vi "Display merged still images.vi"(0 "Image colors":u32[](array[colorbox])=[16711680, 1048329], 3 "Image info":T3(array[cluster])=[{"File name"=path "\\\\jg-i\\c-drive/LabView development/Glimpse/Test Data/Merge test/gelles00096full.tif", "TIFF stack?"=TRUE, "Frame # if stack?"=1}, {"File name"=path "\\\\jg-i\\c-drive/LabView development/Glimpse/Test Data/Merge test/gelles00097full.tif", "TIFF stack?"=TRUE, "Frame # if stack?"=1}], 5 "Transform":u16(ring) items=["linear conformal", "affine", "projective"]) -> (1 "ROI Out":i32[](array[numeric]), 4 "Transform out":u16(ring) items=["linear conformal", "affine", "projective"], 6 "Image info Out":T3(array[cluster])=[{"File name"=path "\\\\jg-i\\c-drive/LabView development/Glimpse/Test Data/Merge test/gelles00096full.tif", "TIFF stack?"=TRUE, "Frame # if stack?"=1}, {"File name"=path "\\\\jg-i\\c-drive/LabView development/Glimpse/Test Data/Merge test/gelles00097full.tif", "TIFF stack?"=TRUE, "Frame # if stack?"=1}], 7 "Display info out":T2(array[cluster]), 8 "Image colors out":u32[](array[colorbox])=[16711680, 1048329])   [LabVIEW 2011]
doc: "Allows the user to select two still images (individual tiffs or frames from a stack) and adust their black/white levels while displaying a pseudocolor merged image. Merged image can optionally be saved as a JPEG file."
uses:
  <vilib>/vision/Image Controls.llb/IMAQ Image.ctl
  GLIMPSE Globals.vi
panel:
  in  "Crop":bool
  in  "Remove\nCrop":bool
  in  "Save\nMerged Image":bool
  in  "Write text overlay":bool=TRUE
  in  "stop":bool
  in  "Load\nimages":bool
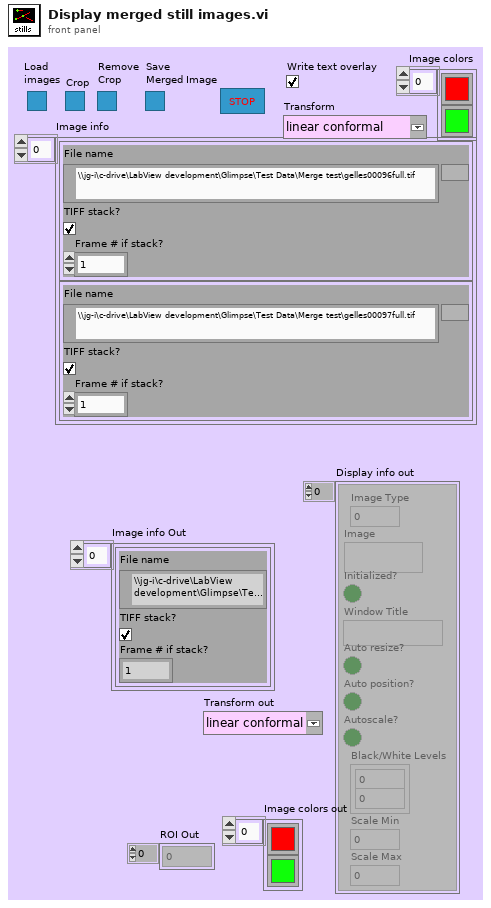
[diagram p1: front panel]
types:
  T1 = typedef "IMAQ Image.ctl" = refnum<image>
  T2 = cluster{"Image Type":u32, "Image":T1, "Initialized?":bool, "Window Title":string, "Auto resize?":bool, "Auto position?":bool, "Autoscale?":bool, "Black/White Levels":cluster{ext, ext}, "Scale Min":ext, "Scale Max":ext}[]
  T3 = cluster{"File name":path, "TIFF stack?":bool, "Frame # if stack?":u32}[]
  T4 = typedef "ROI Descriptor" = cluster{"Global Rectangle":i32[], "Contours":cluster{"ID":enum32{"External", "Internal"}, "Type":u32, "Coordinates":i32[]}[]}
  T5 = enum32{"existing file", "new file", "new or existing file", "existing dir", "new dir", "new or existing dir", "existing file (use LLBs)", "new file (use LLBs)", "new or existing file (use LLBs)", "new or existing file or directory (use LLBs)"}
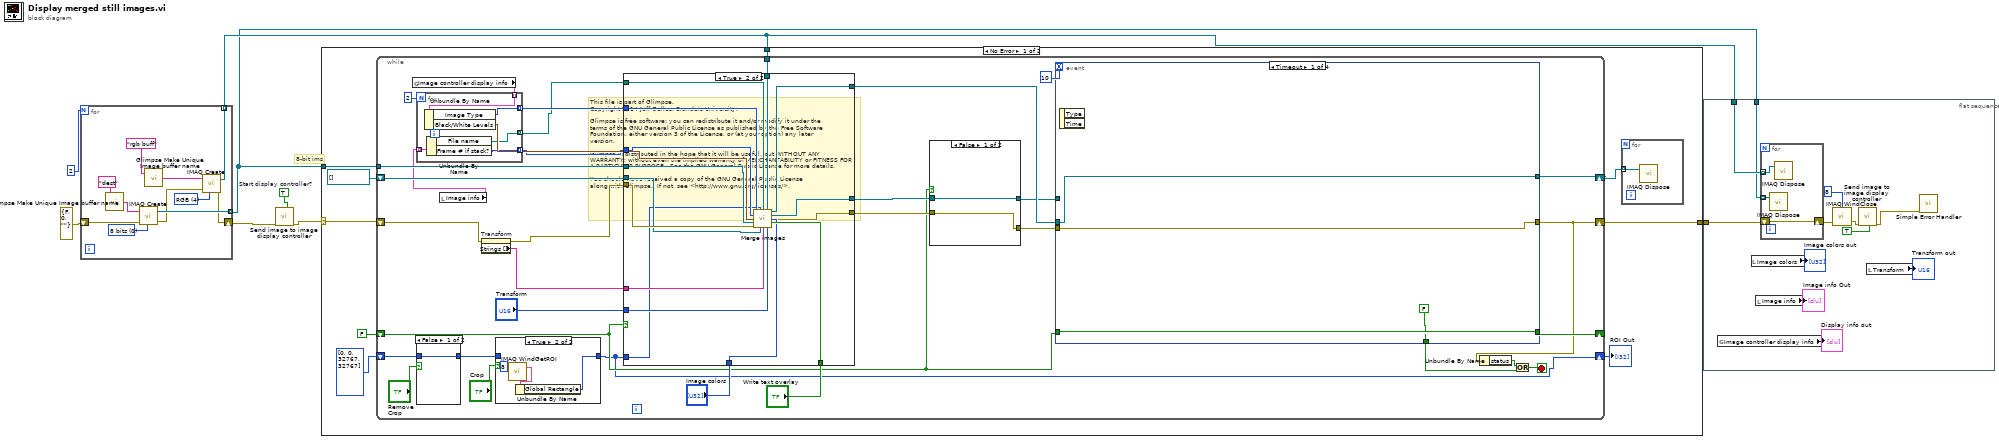
[diagram p0: block diagram]
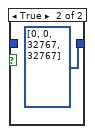
[diagram p3: hidden frame]
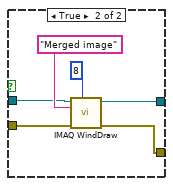
[diagram p4: hidden frame]
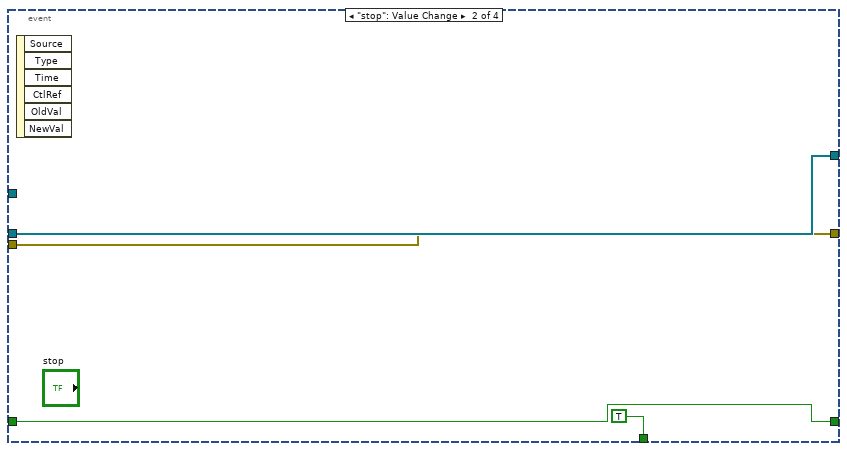
[diagram p6: hidden frame]
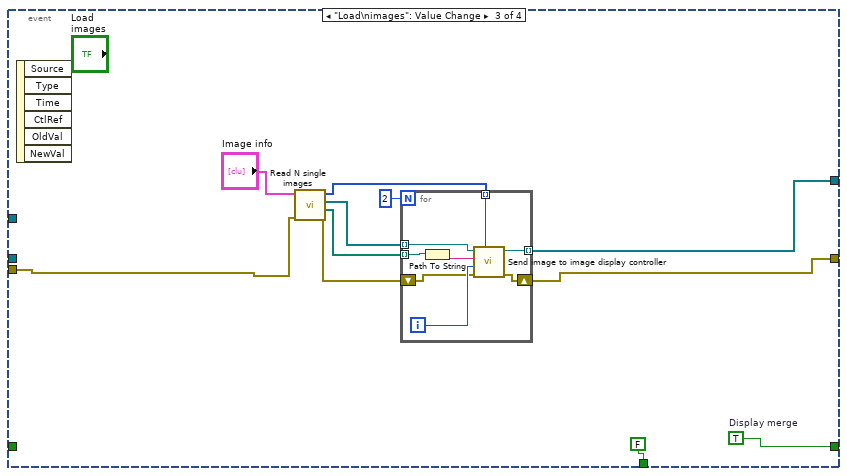
[diagram p7: hidden frame]
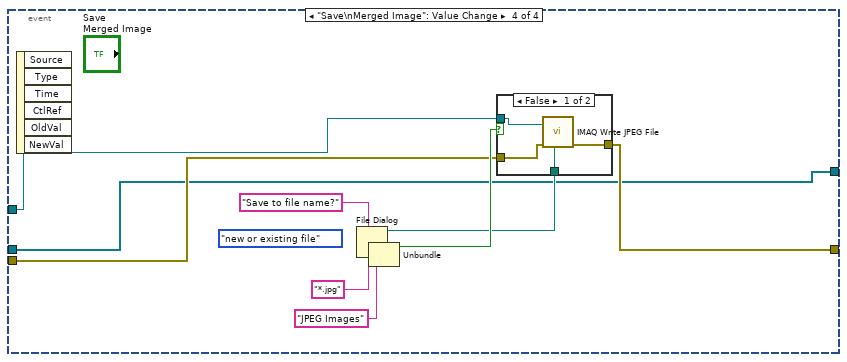
[diagram p8: hidden frame]
diagram:
  w8 = TRUE  # Start display controller?
  # "This file is part of Glimpse. \nCopyright 2014 Jeff Gelles, Brandeis University.    \n\nGlimpse is free software: you can redistribute it and/or modify it under the \nterms of the GNU General Public License as published by the Free Software \nFoundation, either version 3 of the License, or (at your option) any later \nversion.\n\nGlimpse is distributed in the hope that it will be useful, but WITHOUT ANY \nWARRANTY; without even the implied warranty of MERCHANTABILITY or FITNESS FOR \nA PARTICULAR PURPOSE.  See the GNU General Public License for more details.\n\nYou should have received a copy of the GNU General Public License\nalong with Glimpse.  If not, see <http://www.gnu.org/licenses/>."
  # "8-bit ims"
  n1 = for {
    N: 2 -> [_]
    shift-right: [w9] -> w4
    shift-left: errorcluster {"status"=FALSE, "code"=0, "source"=""} ("error out") -> [w16]
    tunnel: [w15] -> w1 mode=indexing
    tunnel: [w13] -> w3 mode=indexing
    w14 = u32 4 items=["8 bits", "16 bits", "Float", "Complex", "RGB", "HSL"] ("Image Type")
    w17 = u32 0 items=["8 bits", "16 bits", "Float", "Complex", "RGB", "HSL"] ("Image Type")
    n2 = call "Glimpse Make Unique Image buffer name.vi"("Buffer  base name"="dest") -> ("Image Name"=w19:string)  [unwired: 1 out]
    n3 = call "IMAQ Create"("Image Name"=w19, "Image Type"=w17, "error in (no error)"=w16) -> ("New Image"=w15:T1, "error out"=w10:errorcluster)  [unwired: 1 in, 1 out]
    n4 = call "Glimpse Make Unique Image buffer name.vi"("Buffer  base name"="rgb buff" ("Image Name")) -> ("Image Name"=w11:string)  [unwired: 1 out]
    n5 = call "IMAQ Create"("Image Name"=w11, "Image Type"=w14, "error in (no error)"=w10) -> ("New Image"=w13:T1, "error out"=w9:errorcluster)  [unwired: 1 in, 1 out]
  }
  n6 = call "Send image to image display controller.vi"("error in"=w4, "Start display controller?"=w8) -> ("error out"=w7:errorcluster)  [unwired: 5 in, 3 out]
  n7 = case shown="No Error" w7 {
    selector: w7 -> [w27 _]
    tunnel: w1 -> [w26 _]
    tunnel: w3 -> [w25 _]
    tunnel: [w23 _] -> w2
    frame No Error {
      n8 = while {
        shift-right: [w63] -> _
        shift-left: FALSE ("Display merge") -> [w40]
        shift-right: [w57] -> w23
        shift-left: w27 -> [w37]
        tunnel: w26 -> [w62]
        shift-right: [w61] -> w24
        shift-left: T1[] [] -> [w60]
        tunnel: w25 -> [w59]
        shift-right: [w30] -> w20
        shift-left: i32[] [0, 0, 32767, 32767] ("ROI") -> [w32]
        stop <- w54 stop-if-true
        n9 = global read "GLIMPSE Globals.vi" "Image controller display info"() -> (w51:T2)
        n10 = case shown="False" "Remove\nCrop" {
          tunnel: w32 -> [w68 _]
          tunnel: [w68 i32[] [0, 0, 32767, 32767] ("ROI")] -> w31
          frame False {
          }
          frame True {
          }
        }
        n11 = local read "Image info"() -> (w47:T3)
        n12 = for {
          N: 2 -> [_]
          tunnel: w51 -> [w83] mode=indexing
          tunnel: [w82] -> w50 mode=indexing
          tunnel: [w81] -> w48 mode=indexing
          tunnel: [w78] -> w49 mode=indexing
          tunnel: w47 -> [w80] mode=indexing
          tunnel: [w79] -> w46 mode=indexing
          n13 = Unbundle By Name(w83) -> ("Image Type"=w82:u32, "Black/White Levels"=w81:cluster{ext, ext})
          n14 = Unbundle By Name(w80) -> ("File name"=w78:path, "Frame # if stack?"=w79:u32)
        }
        n15 = property on="Transform" class="Ring (strict)"(error in=w37) -> (error out=w36:errorcluster, "Strings []"=w38:string[])  [unwired: 1 in, 1 out]
        n16 = case shown="True" "Crop" {
          tunnel: w31 -> [w64 _]
          tunnel: [w64 w65] -> w30
          frame False {
          }
          frame True {
            n17 = call "IMAQ WindGetROI"("Window Number (0...15)"=8) -> ("ROI Descriptor"=w67:T4)  [unwired: 1 in, 4 out]
            n18 = Unbundle By Name(w67) -> ("Global Rectangle"=w65:i32[])
          }
        }
        n19 = case shown="True" w40 {
          tunnel: w62 -> [_ w101]
          tunnel: w36 -> [w84 w100]
          tunnel: w60 -> [w85 w99]
          tunnel: w59 -> [_ w98]
          tunnel: [w84 w90] -> w43
          tunnel: [w85 w97] -> w58
          tunnel: w50 -> [_ w96]
          tunnel: w48 -> [_ w95]
          tunnel: w49 -> [_ w94]
          tunnel: w46 -> [_ w93]
          tunnel: "Write text overlay" -> [_ w92]
          tunnel: "Image colors" -> [_ w91]
          tunnel: [_ w89] -> w41
          tunnel: "Transform" -> [_ w88]
          tunnel: w38 -> [_ w87]
          tunnel: w30 -> [_ w86]
          frame False {
          }
          frame True {
            n20 = call "Merge images.vi"("Image types"=w96, "ROI"=w86, "File paths"=w94, "RGB image buffers in"=w98, "Overlay frame numbers"=w93, "Black/white levels"=w95, "8 bit scratch images"=w101, "Write text overlay?"=w92, "error in"=w100, "N-bit images in"=w99, "Transform types"=w87, "Transform number?"=w88, "Image colors"=w91) -> ("N-bit images out"=w97:T1[], "RGB Image out"=w89:T1, "error out"=w90:errorcluster)
          }
        }
        n21 = case shown="False" w40 {
          tunnel: w43 -> [w71 w75]
          tunnel: [w71 w74] -> w42
          tunnel: w41 -> [w70 w73]
          tunnel: [w70 w72] -> w35
          frame False {
          }
          frame True {
            n22 = call "IMAQ WindDraw"("Window Number (0...15)"=8, "error in (no error)"=w75, "Title"="Merged image", "Image"=w73) -> ("error out"=w74:errorcluster, "Image Out (duplicate)"=w72:T1)  [unwired: 2 in, 4 out]
          }
        }
        n23 = event shown="[0] Timeout" {
          selector: _ -> [_ _ _ _]
          dyn-events: _ -> [_ _ _ _]
          timeout: 10 -> [_ _ _ _]
          tunnel: [w104 w106 w115 _] -> w63
          tunnel: w40 -> [w104 w106 _ _]
          tunnel: [w105 w108 w114 w130] -> w61
          tunnel: w58 -> [w105 w108 _ w130]
          tunnel: [w103 w107 w110 w131] -> w57
          tunnel: w42 -> [w103 w107 w111 w132]
          tunnel: [FALSE TRUE FALSE _] -> w55
          tunnel: w35 -> [_ _ _ w133]
          event Timeout {
            n24 = event-data() -> ()  [unwired: 3 out]
          }
          event "stop": Value Change {
            n25 = event-data() -> ()  [unwired: 7 out]
          }
          event "Load\nimages": Value Change {
            w115 = TRUE  # Display merge
            n26 = event-data() -> ()  [unwired: 7 out]
            n27 = call "Read N single images.vi"("error in"=w111, "Image info"="Image info") -> ("error out"=w119:errorcluster, "File paths out"=w118:path[], "Images out"=w117:T1[], "Image types out"=w116:u32[])  [unwired: 4 out]
            n28 = for {
              N: 2 -> [_]
              tunnel: [w127] -> w114 mode=indexing
              shift-right: [w126] -> w110
              shift-left: w119 -> [w122]
              tunnel: w118 -> [w124] mode=indexing
              tunnel: w117 -> [w123] mode=indexing
              tunnel: w116 -> [w121] mode=indexing
              i -> [w125]
              n29 = Path To String(path=w124) -> (string=w128:string)
              n30 = call "Send image to image display controller.vi"("Image"=w123, "Window Title"=w128, "Window Number"=w125, "error in"=w122, "Image Type"=w121) -> ("Image Out"=w127:T1, "error out"=w126:errorcluster)  [unwired: 2 in, 2 out]
            }
          }
          event "Save\nMerged Image": Value Change {
            (unwired) T5."new or existing file" ("select mode (2)")
            n31 = event-data() -> ()  [unwired: 7 out]
            n32 = File Dialog(4:"JPEG Images" ("pattern label"), 6:"*.jpg" ("pattern"), 7:"Save to file name?" ("prompt")) -> (0:w129:errorcluster, 1:w138:bool, 3:w137:path)  [unwired: 1 in, 4 out]
            n33 = Unbundle(w129) -> ()  [unwired: 3 out]
            n34 = case shown="False" w138 {
              tunnel: [w142 w143] -> w131
              tunnel: w132 -> [w141 w143]
              tunnel: w137 -> [w140 _]
              tunnel: w133 -> [w139 _]
              frame False {
                n35 = call "IMAQ Write JPEG File"("error in (no error)"=w141, "File Path"=w140, "Image"=w139) -> ("error out"=w142:errorcluster)  [unwired: 2 in, 3 out]
              }
              frame True {
              }
            }
          }
        }
        n36 = Unbundle By Name(w57) -> ("status"=w56:bool)
        n37 = Or(x=w56, y=w55) -> (x .or. y?=w54:bool)
      }
      "ROI Out" <- w20
      n38 = for {
        tunnel: w24 -> [w29] mode=indexing
        n39 = call "IMAQ Dispose"("Image"=w29) -> ()  [unwired: 2 in, 4 out]
      }
    }
    frame Error {
    }
  }
  n40 = flat-sequence {
    tunnel: w3 -> [w155]
    tunnel: w2 -> [w154]
    tunnel: w1 -> [w153]
    frame #0 {
      n41 = global read "GLIMPSE Globals.vi" "Image controller display info"() -> (→"Display info out":T2)
      n42 = local read "Image colors"() -> (→"Image colors out":u32[])
      n43 = local read "Image info"() -> (→"Image info Out":T3)
      n44 = for {
        tunnel: w155 -> [w157] mode=indexing
        shift-right: [w158] -> w152
        shift-left: w154 -> [w158]
        tunnel: w153 -> [w156] mode=indexing
        n45 = call "IMAQ Dispose"("Image"=w156) -> ()  [unwired: 2 in, 4 out]
        n46 = call "IMAQ Dispose"("Image"=w157) -> ()  [unwired: 2 in, 4 out]
      }
      n47 = call "IMAQ WindClose"("Window Number (0...15)"=8, "error in (no error)"=w152) -> ("error out"=w151:errorcluster)  [unwired: 1 in, 3 out]
      n48 = call "Send image to image display controller.vi"("error in"=w151, "Quit display controller?"=TRUE) -> ("error out"=w150:errorcluster)  [unwired: 5 in, 3 out]
      n49 = local read "Transform"() -> (→"Transform out":u16)
      n50 = call <vilib>:"Simple Error Handler.vi"("error in (no error)"=w150) -> ()  [unwired: 1 in, 8 out]
    }
  }
